vi "Run Tests.vi"() -> ()   [LabVIEW 2019, in "RESP3 Tests.lvlib"]
uses:
  RESP3 Tests.lvlib
  <vilib>/Utility/miscctls.llb/LVRowAndColumnTypeDef.ctl
  <vilib>/Analysis/baseanly.llb/Mean (DBL).vi
  <vilib>/regexp/Match Regular Expression.xnode
  <vilib>/ptbypt/NI_PtbyPt.lvlib
  <vilib>/gmath/NI_Gmath.lvlib
  <vilib>/Analysis/NI_AALBase.lvlib
panel:
  in  "max iters per":i32=25
  out "current test":string
  out "Test Results":string[][](table)
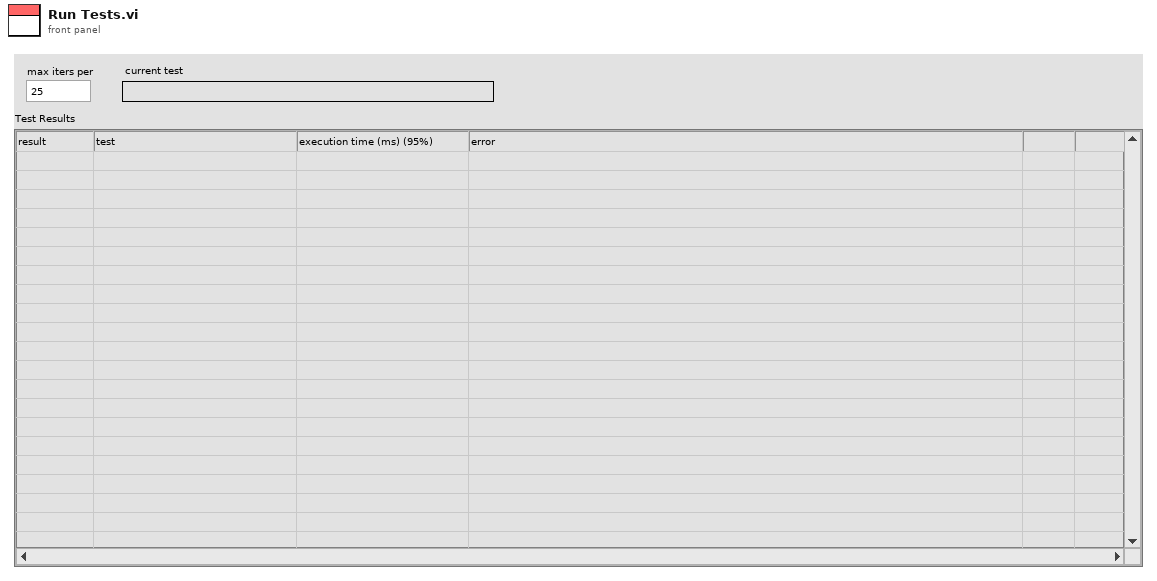
[diagram p1: front panel]
types:
  T1 = typedef "LVRowAndColumnTypeDef.ctl" = cluster{"Row":i32, "Column":i32}
  T2 = cluster{string, "pass?":bool, "error IO":errorcluster, "mean":dbl, "confidence interval":cluster{"low":dbl, "high":dbl}}
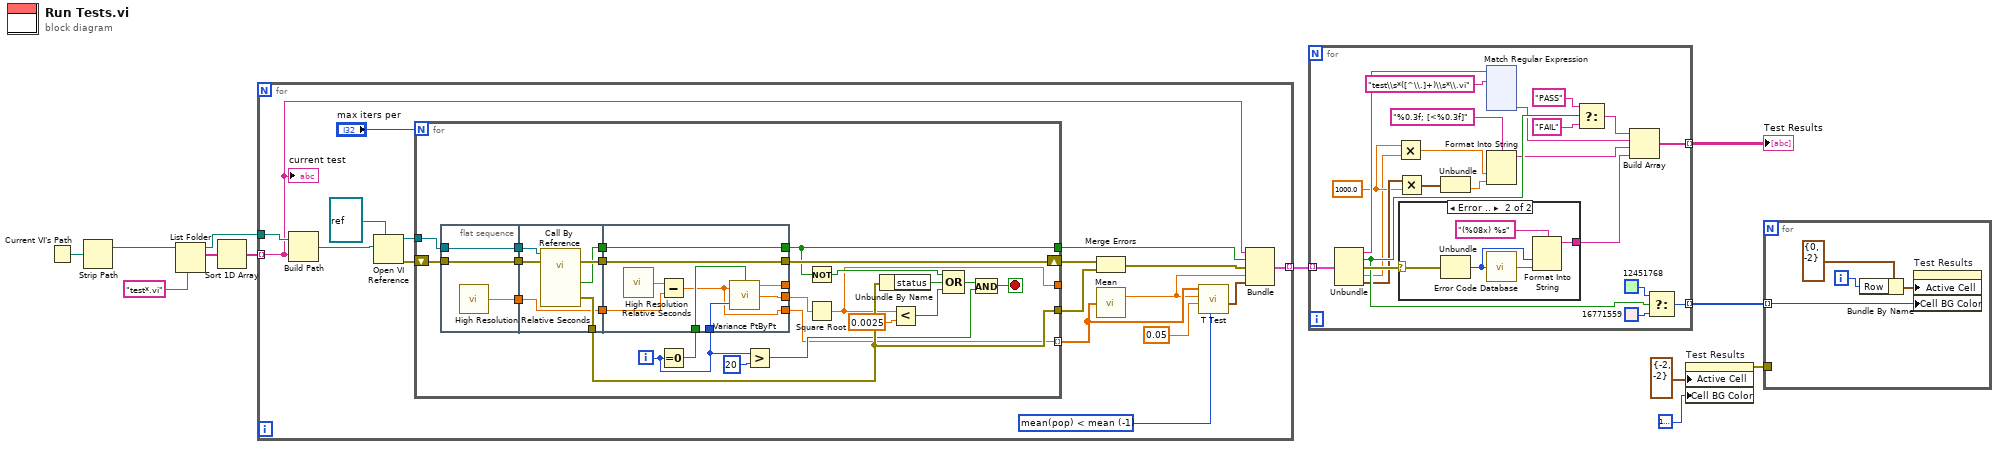
[diagram p0: block diagram]
diagram:
  n1 = Current VI's Path() -> (path=w12:path)
  n2 = Strip Path(path=w12) -> (stripped path=w11:path)  [unwired: 1 out]
  n3 = List Folder(path=w11, pattern="test*.vi") -> (path out=w7:path, filenames=w9:string[])  [unwired: 2 in, 2 out]
  n4 = Sort 1D Array(array=w9) -> (sorted array=w8:string[])
  n5 = for {
    tunnel: w8 -> [w19] mode=indexing
    tunnel: w7 -> [w28]
    tunnel: [w20] -> w6 mode=indexing
    w15 = -1 items=["mean(pop) != mean"=0, "mean(pop) > mean"=1, "mean(pop) < mean"=-1] ("alternative hypothesis")
    n6 = Build Path(base path=w28, name or relative path=w19) -> (appended path=w27:path)
    n7 = Open VI Reference(type specifier VI Refnum (for type only)=refnum<vi> refnum, vi path=w27) -> (vi reference=w26:refnum<vi>, error out=w25:errorcluster)  [unwired: 4 in]
    n8 = for {
      N: "max iters per" -> [_]
      tunnel: w26 -> [w53]
      tunnel: [w50] -> w23
      tunnel: [w48] -> w22
      shift-right: [w51] -> w24
      shift-left: w25 -> [w52]
      tunnel: [w31] -> _
      tunnel: [w30] -> w17 mode=indexing
      i -> [w36]
      stop <- w34 stop-if-true
      n9 = flat-sequence {
        tunnel: w52 -> [w55]
        tunnel: w53 -> [w56]
        tunnel: [w56] -> w43
        tunnel: [w55] -> w42
        tunnel: [w54] -> w41
        tunnel: [w59] -> w50
        tunnel: [w60] -> w45
        tunnel: [w58] -> w44
        tunnel: w43 -> [w62]
        tunnel: w42 -> [w61]
        tunnel: w41 -> [w57]
        tunnel: [w57] -> w40
        tunnel: [w70] -> w48
        tunnel: [w71] -> w51
        tunnel: w45 -> [w71]
        tunnel: w44 -> [w70]
        tunnel: w40 -> [w68]
        tunnel: w39 -> [w67]
        tunnel: w36 -> [w66]
        tunnel: [w65] -> _
        tunnel: [w64] -> w32
        tunnel: [w63] -> w30
        frame #0 {
          n10 = call <vilib>:"High Resolution Relative Seconds.vi"() -> ("relative seconds"=w54:dbl)
        }
        frame #1 {
          n11 = call-by-ref "?"(reference=w62, error in=w61) -> (error out=w60:errorcluster, 0:"error out"=w59:errorcluster, "pass?"=w58:bool)  [unwired: 10 in, 1 out]
        }
        frame #2 {
          n12 = call <vilib>:"High Resolution Relative Seconds.vi"() -> ("relative seconds"=w69:dbl)
          n13 = Subtract(x=w69, y=w68) -> (x-y=w63:dbl)
          n14 = call <vilib>:"Variance PtByPt.vi"("x"=w63, "sample length"=w66, "initialize"=w67) -> ("mean"=w65:dbl, "variance"=w64:dbl)  [unwired: 1 out]
        }
      }
      n15 = Equal To 0?(x=w36) -> (x = 0?=w39:bool)
      n16 = Greater?(x=w36, y=20) -> (0:w33:bool)
      n17 = Not(x=w48) -> (.not. x?=w47:bool)
      n18 = Square Root(x=w32) -> (sqrt(x)=w31:dbl)
      n19 = Unbundle By Name(w50) -> ("status"=w49:bool)
      n20 = Less?(x=w31, y=0.0025) -> (x < y?=w37:bool)
      n21 = Compound Arithmetic op=OR(w47, w49, w37) -> (w46:bool)
      n22 = Compound Arithmetic op=AND(w46, w33) -> (w34:bool)
    }
    n23 = Merge Errors(w24, w23) -> (w21:errorcluster)
    n24 = call-poly <vilib>:"Mean.vi"("X"=w17) -> ("mean"=w13:dbl)  [unwired: 1 out]
    n25 = call <vilib>:"T Test.vi"("alternative hypothesis"=w15, "significance level"=0.05, "mean"=w13, "sample set"=w17) -> ("confidence interval"=w14:cluster{"low":dbl, "high":dbl})  [unwired: 3 in, 4 out]
    n26 = Bundle(w19, "pass?"=w22, "error IO"=w21, "mean"=w13, "confidence interval"=w14) -> (w20:T2)  [unwired: 1 in]
    "current test" <- w19
  }
  n27 = for {
    tunnel: w6 -> [w93] mode=indexing
    tunnel: [w86] -> w5 mode=indexing
    tunnel: [w84] -> w4 mode=indexing
    w74 = 1000.0 ("y")
    n28 = Unbundle(w93) -> (w82:string, "pass?"=w89:bool, "error IO"=w90:errorcluster, "mean"=w73:dbl, "confidence interval"=w77:cluster{"low":dbl, "high":dbl})
    n29 = Multiply(x=w74, y=w73) -> (x*y=w72:dbl)
    n30 = Multiply(x=w77, y=w74) -> (x*y=w76:cluster{"low":dbl, "high":dbl})
    n31 = case shown="Error .." w90 {
      selector: w90 -> [_ w212]
      tunnel: [_ w213] -> w80
      frame No Error {
      }
      frame Error {
        n32 = Unbundle(w212) -> ("code"=w211:i32)  [unwired: 2 out]
        n33 = call <vilib>:"Error Code Database.vi"("Error Code"=w211) -> ("Error Text"=w210:string)
        n34 = Format Into String(format string="(%08x) %s", w211, w210) -> (resulting string=w213:string)  [unwired: 2 in, 1 out]
      }
    }
    n35 = Unbundle(w76) -> ("high"=w75:dbl)  [unwired: 1 out]
    n36 = xnode "Match Regular Expression"("input string"=w82, "regular expression"="test\\s*([^\\.]+)\\s*\\.vi") -> ("submatch 1"=w81:string)  [unwired: 4 in, 5 out]
    n37 = Format Into String(format string="%0.3f; [<%0.3f]", w72, w75) -> (resulting string=w78:string)  [unwired: 2 in, 1 out]
    n38 = Select(t="PASS", s=w89, f="FAIL") -> (s? t:f=w85:string)
    n39 = Build Array(w85, w81, w78, w80) -> (w86:string[])
    n40 = Select(t=u32 12451768, s=w89, f=u32 16771559) -> (s? t:f=w84:u32)
  }
  "Test Results" <- w5
  n41 = property on="Test Results" class="Tbl (strict)"("Active Cell"=T1 {"Row"=-2, "Column"=-2} ("Active Cell:Active Cell"), "Cell BG Color"=u32 16777225 ("Active Cell:Cell Background Color")) -> (error out=w3:errorcluster)  [unwired: 2 in, 1 out]
  n42 = for {
    tunnel: w4 -> [w215] mode=indexing
    tunnel: w3 -> [_]
    i -> [w217]
    n43 = Bundle By Name(cluster=T1 {"Row"=0, "Column"=-2} ("Active Cell:Active Cell"), "Row"=w217) -> (w216:T1)
    n44 = property on="Test Results" class="Tbl (strict)"("Active Cell"=w216, "Cell BG Color"=w215) -> ()  [unwired: 2 in, 2 out]
  }
